vi "Planck.vi"(1 "Wavelength (µm)":dbl=9.5, 2 "Temperature (K)":dbl=288.0) -> (0 "Spectral emittance (W m-2 µm-1)":dbl[unit]=8.050830230935293)   [LabVIEW 2012]
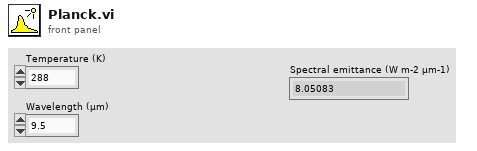
[diagram p1: front panel]
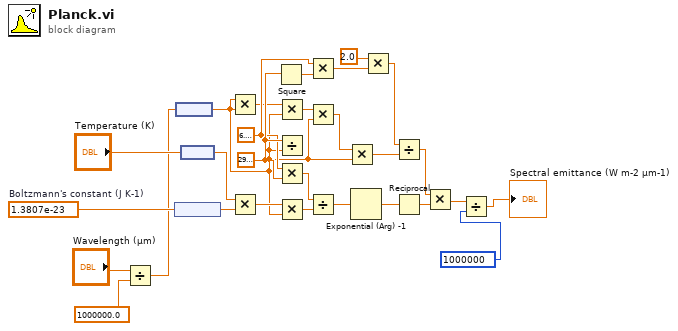
[diagram p0: block diagram]
diagram:
  w17 = dbl[unit] 6.6260693e-34
  w19 = dbl[unit] 299792458.0
  w23 = 1.3807e-23  # Boltzmann's constant (J K-1)
  n1 = Divide(x="Wavelength (µm)", y=1000000.0) -> (x/y=w6:dbl)
  n2 = node(w23) -> (w22:dbl[unit])
  n3 = node(w6) -> (w11:dbl[unit])
  n4 = node("Temperature (K)") -> (w24:dbl[unit])
  n5 = Multiply(x=w11, y=w11) -> (x*y=w14:dbl[unit])
  n6 = Multiply(x=w24, y=w22) -> (x*y=w26:dbl[unit])
  n7 = Square(x=w19) -> (x^2=w18:dbl[unit])
  n8 = Multiply(x=w14, y=w11) -> (x*y=w13:dbl[unit])
  n9 = Divide(x=w19, y=w11) -> ()  [unwired: 1 out]
  n10 = Multiply(x=w17, y=w19) -> (x*y=w28:dbl[unit])
  n11 = Multiply(x=w26, y=w11) -> (x*y=w27:dbl[unit])
  n12 = Multiply(x=w17, y=w18) -> (x*y=w16:dbl[unit])
  n13 = Multiply(x=w13, y=w11) -> (x*y=w12:dbl[unit])
  n14 = Divide(x=w28, y=w27) -> (x/y=w21:dbl)
  n15 = Multiply(x=w12, y=w11) -> (x*y=w9:dbl[unit])
  n16 = Exponential (Arg) -1(1:w21) -> (0:w20:dbl)
  n17 = Multiply(x=2.0, y=w16) -> (x*y=w10:dbl[unit])
  n18 = Divide(x=w10, y=w9) -> (x/y=w8:dbl[unit])
  n19 = Reciprocal(x=w20) -> (1/x=w7:dbl)
  n20 = Multiply(x=w8, y=w7) -> (x*y=w2:dbl[unit])
  n21 = Divide(x=w2, y=1000000) -> (x/y=→"Spectral emittance (W m-2 µm-1)":dbl[unit])
